vi "Globals.vi"() -> ()   [LabVIEW 2020, in "SMCD14_lib.lvlib"]
uses:
  SMCD14_lib.lvlib
  ConnectionData_typedef.ctl
  <vilib>/Modbus/master/Modbus Master.lvclass
  <vilib>/Modbus/subvis/Transmission Data Unit (ADU)/RTU Data Unit/RTU Data Unit.lvclass
  <vilib>/Modbus/subvis/Protocol/Serial/Serial Master/Serial Master.lvclass
  AxisConfiguration_typedef.ctl
  AxisWriteValues_typedef.ctl
  AxisReadValues_typedef.ctl
panel:
  in  "AxisReadValues":T1[](array[typedef])
  in  "AxisWriteValues":T2[](array[typedef])=[{"AxisTarget"=0.0, "AxisTargetVel"=1.0, "AxisStartReq"=FALSE, "AxisStopReq"=FALSE, "AxisClearReq"=FALSE, "AxisMovetype"=FALSE, "AxisMotorON"=FALSE, "MoveModeControl"=0, "AxisHomingVel"=1.0, "AxisAccDecc"=30.0}, {"AxisTarget"=0.0, "AxisTargetVel"=1.0, "AxisStartReq"=FALSE, "AxisStopReq"=FALSE, "AxisClearReq"=FALSE, "AxisMovetype"=FALSE, "AxisMotorON"=FALSE, "MoveModeControl"=0, "AxisHomingVel"=1.0, "AxisAccDecc"=30.0}, {"AxisTarget"=0.0, "AxisTargetVel"=1.0, "AxisStartReq"=FALSE, "AxisStopReq"=FALSE, "AxisClearReq"=FALSE, "AxisMovetype"=FALSE, "AxisMotorON"=FALSE, "MoveModeControl"=0, "AxisHomingVel"=1.0, "AxisAccDecc"=30.0}, {"AxisTarget"=0.0, "AxisTargetVel"=1.0, "AxisStartReq"=FALSE, "AxisStopReq"=FALSE, "AxisClearReq"=FALSE, "AxisMovetype"=FALSE, "AxisMotorON"=FALSE, "MoveModeControl"=0, "AxisHomingVel"=1.0, "AxisAccDecc"=30.0}, {"AxisTarget"=0.0, "AxisTargetVel"=1.0, "AxisStartReq"=FALSE, "AxisStopReq"=FALSE, "AxisClearReq"=FALSE, "AxisMovetype"=FALSE, "AxisMotorON"=FALSE, "MoveModeControl"=0, "AxisHomingVel"=1.0, "AxisAccDecc"=30.0}, {"AxisTarget"=0.0, "AxisTargetVel"=1.0, "AxisStartReq"=FALSE, "AxisStopReq"=FALSE, "AxisClearReq"=FALSE, "AxisMovetype"=FALSE, "AxisMotorON"=FALSE, "MoveModeControl"=0, "AxisHomingVel"=1.0, "AxisAccDecc"=30.0}] {"MoveModeControl" items=["Absolute"=1, "Relative"=2, "Velocity"=3, "Homing"=4, "none"=0]}
  in  "AxisConfiguration":T3[](array[typedef])=[{"AxisHomeType"=1, "AxisBacklash"=0.0, "AxisGain"=1.0, "AxisOffset"=0.0, "AxisUnit"=0, "ReqConfRead"=FALSE, "ReqConfWrite"=FALSE, "AxisName"="", "AxisAccDecc"=0.0, "AxisHomeVel"=0.0}, {"AxisHomeType"=1, "AxisBacklash"=0.0, "AxisGain"=1.0, "AxisOffset"=0.0, "AxisUnit"=0, "ReqConfRead"=FALSE, "ReqConfWrite"=FALSE, "AxisName"="", "AxisAccDecc"=0.0, "AxisHomeVel"=0.0}, {"AxisHomeType"=1, "AxisBacklash"=0.0, "AxisGain"=1.0, "AxisOffset"=0.0, "AxisUnit"=0, "ReqConfRead"=FALSE, "ReqConfWrite"=FALSE, "AxisName"="", "AxisAccDecc"=0.0, "AxisHomeVel"=0.0}, {"AxisHomeType"=1, "AxisBacklash"=0.0, "AxisGain"=1.0, "AxisOffset"=0.0, "AxisUnit"=0, "ReqConfRead"=FALSE, "ReqConfWrite"=FALSE, "AxisName"="", "AxisAccDecc"=0.0, "AxisHomeVel"=0.0}, {"AxisHomeType"=1, "AxisBacklash"=0.0, "AxisGain"=1.0, "AxisOffset"=0.0, "AxisUnit"=0, "ReqConfRead"=FALSE, "ReqConfWrite"=FALSE, "AxisName"="", "AxisAccDecc"=0.0, "AxisHomeVel"=0.0}, {"AxisHomeType"=1, "AxisBacklash"=0.0, "AxisGain"=1.0, "AxisOffset"=0.0, "AxisUnit"=0, "ReqConfRead"=FALSE, "ReqConfWrite"=FALSE, "AxisName"="", "AxisAccDecc"=0.0, "AxisHomeVel"=0.0}] {"AxisUnit" items=["mm", "°"]; "AxisHomeType" items=["no homing"=0, "forward limit switch"=1, "backward limit switch"=2, "forward reference"=4, "backward reference"=8]}
  in  "ConnectionData":T4[](array[typedef])=[{"DeviceIDCtrl"=1, "ProtocolCtrl"=enum."Modbus RTU", "COMportCtrl"="COM2", "IPCtrl"="", "serial master instance"=refnum, "ConnectionStatusIndicator"=FALSE}, {"DeviceIDCtrl"=1, "ProtocolCtrl"=enum."Modbus RTU", "COMportCtrl"="COM2", "IPCtrl"="", "serial master instance"=refnum, "ConnectionStatusIndicator"=FALSE}, {"DeviceIDCtrl"=1, "ProtocolCtrl"=enum."Modbus RTU", "COMportCtrl"="COM2", "IPCtrl"="", "serial master instance"=refnum, "ConnectionStatusIndicator"=FALSE}, {"DeviceIDCtrl"=1, "ProtocolCtrl"=enum."Modbus RTU", "COMportCtrl"="COM2", "IPCtrl"="", "serial master instance"=refnum, "ConnectionStatusIndicator"=FALSE}, {"DeviceIDCtrl"=1, "ProtocolCtrl"=enum."Modbus RTU", "COMportCtrl"="COM2", "IPCtrl"="", "serial master instance"=refnum, "ConnectionStatusIndicator"=FALSE}, {"DeviceIDCtrl"=1, "ProtocolCtrl"=enum."Modbus RTU", "COMportCtrl"="COM2", "IPCtrl"="", "serial master instance"=refnum, "ConnectionStatusIndicator"=FALSE}]
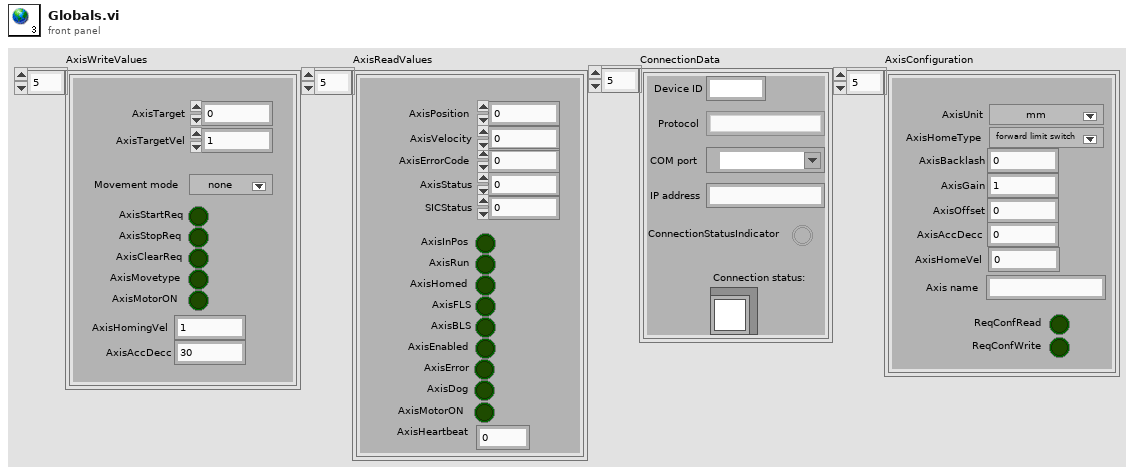
[diagram p1: front panel]
types:
  T1 = typedef "SMCD14_lib.lvlib/AxisReadValues_typedef.ctl" = cluster{"AxisPosition":dbl, "AxisStatus":i16, "AxisErrorCode":i16, "AxisInPos":bool, "AxisRun":bool, "AxisHomed":bool, "AxisFLS":bool, "AxisBLS":bool, "AxisEnabled":bool, "AxisError":bool, "AxisDog":bool, "AxisVelocity":dbl, "AxisHeartbeat":i16, "SICStatus":i16, "AxisMotorON":bool}
  T2 = typedef "SMCD14_lib.lvlib/AxisWriteValues_typedef.ctl" = cluster{"AxisTarget":dbl, "AxisTargetVel":dbl, "AxisStartReq":bool, "AxisStopReq":bool, "AxisClearReq":bool, "AxisMovetype":bool, "AxisMotorON":bool, "MoveModeControl":u16, "AxisHomingVel":dbl, "AxisAccDecc":dbl}
  T3 = typedef "SMCD14_lib.lvlib/AxisConfiguration_typedef.ctl" = cluster{"AxisHomeType":u16, "AxisBacklash":dbl, "AxisGain":dbl, "AxisOffset":dbl, "AxisUnit":u16, "ReqConfRead":bool, "ReqConfWrite":bool, "AxisName":string, "AxisAccDecc":dbl, "AxisHomeVel":dbl}
  T4 = typedef "SMCD14_lib.lvlib/ConnectionData_typedef.ctl" = cluster{"DeviceIDCtrl":u16, "ProtocolCtrl":enum16{"Modbus RTU", "Modbus TCP", ""}, "COMportCtrl":refnum<visa-resource-name>, "IPCtrl":string, "serial master instance":refnum<class "Modbus Master.lvclass">, "ConnectionStatusIndicator":bool}
diagram:
